vi "ManuScanTest.vi"() -> ()   [LabVIEW 2014]
panel:
  out "before substring":string
  out "x = y?":bool
  in  "Key Focus":bool
  in  "stop":bool
  in  "String 2":string
  in  "String":string
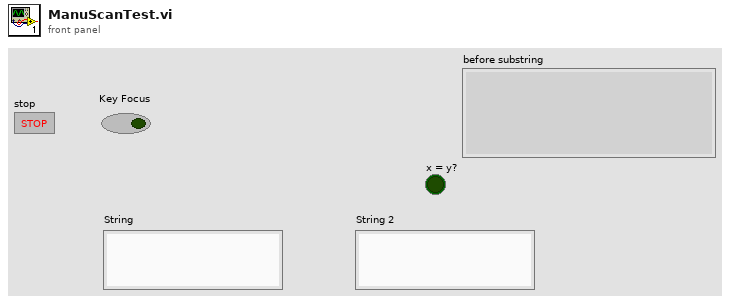
[diagram p1: front panel]
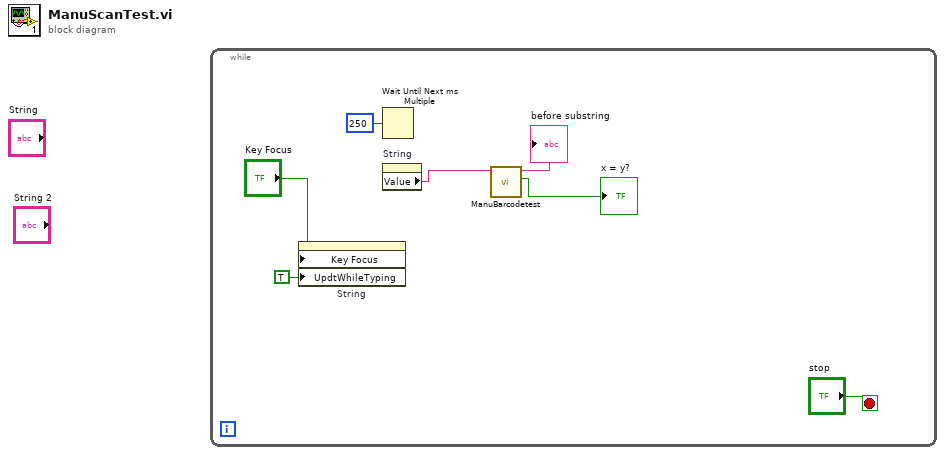
[diagram p0: block diagram]
diagram:
  n1 = while {
    stop <- "stop" stop-if-true
    n2 = property on="String" class="Str"("Key Focus"="Key Focus", "UpdtWhileTyping"=TRUE ("Update While Typing?")) -> ()  [unwired: 2 in, 2 out]
    n3 = Wait Until Next ms Multiple(millisecond multiple=u32 250) -> ()  [unwired: 1 out]
    n4 = property on="String" class="Str"() -> ("Value"=w1:string)  [unwired: 2 in, 2 out]
    n5 = call "ManuBarcodetest.vi"("String"=w1) -> ("x = y?"=→"x = y?":bool, "before substring"=→"before substring":string)  [unwired: 9 in]
  }
